vi "BuildWindowsTarget.vi"(8 "error in (no error)":errorcluster, 11 "Library Builder in":refnum<class "Library Builder.lvclass">) -> (0 "error out":errorcluster, 3 "Library Builder out":refnum<class "Library Builder.lvclass">)   [LabVIEW 2020, in "Library Builder.lvclass"]
uses:
  Library Builder.lvclass
  Library Builder.lvclass/Library Builder.ctl
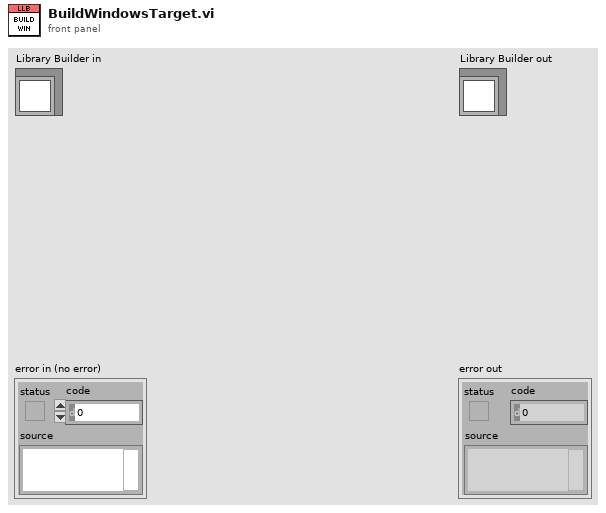
[diagram p1: front panel]
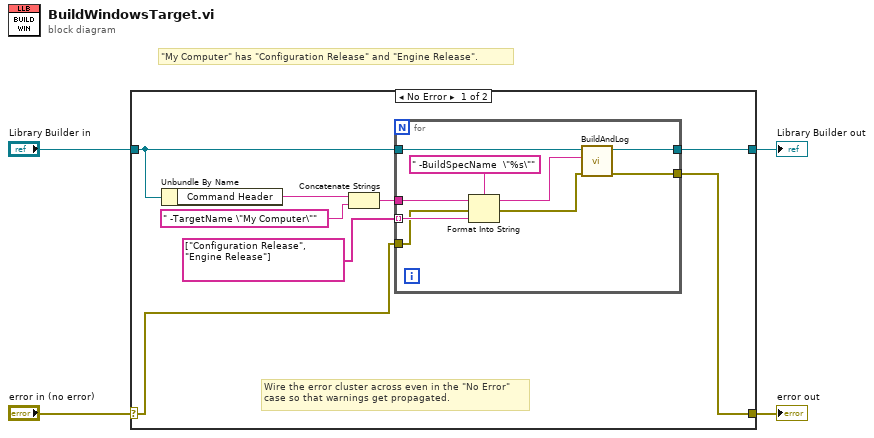
[diagram p0: block diagram]
diagram:
  # "\"My Computer\" has \"Configuration Release\" and \"Engine Release\"."
  n1 = case shown="No Error" "error in (no error)" {
    selector: "error in (no error)" -> [w5 w23]
    tunnel: [w11 w23] -> w3
    tunnel: [w12 w22] -> w1
    tunnel: "Library Builder in" -> [w10 w22]
    frame No Error {
      # "Wire the error cluster across even in the \"No Error\"\ncase so that warnings get propagated."
      n2 = Unbundle By Name(w10) -> ("Command Header"=w9:string)
      n3 = Concatenate Strings(w9, " -TargetName \"My Computer\"") -> (w7:string)
      n4 = for {
        tunnel: [w20] -> w11
        tunnel: w10 -> [w19]
        tunnel: [w21] -> w12
        tunnel: w7 -> [w17]
        tunnel: string[] ["Configuration Release", "Engine Release"] -> [w16] mode=indexing
        tunnel: w5 -> [w15]
        n5 = Format Into String(format string=" -BuildSpecName  \"%s\"", initial string=w17, error in=w15, w16) -> (resulting string=w14:string, error out=w13:errorcluster)
        n6 = call "BuildAndLog.vi"("error in (no error)"=w13, "Command In"=w14, "Library Builder in"=w19) -> ("error out"=w20:errorcluster, "Library Builder out"=w21:refnum<class "Library Builder.lvclass">)  [unwired: 7 in]
      }
    }
    frame Error {
    }
  }
  "error out" <- w3
  "Library Builder out" <- w1
